vi "CCSaveWorklistResult.vi"(8 "error in (no error)":errorcluster, 9 "patientID":string="C:\\Users\\Simon\\Dropbox\\Medimatic\\ProjectVerLV2011\\tmp.dcm", 10 "index":i32, 11 "Find":refnum<k24>) -> (0 "error out":errorcluster)   [LabVIEW 2013, in "main.lvlib" / "ClearCanvasLibrary.lvlib"]
uses:
  ClearCanvasLibrary.lvlib
  C:/Users/Simon/SkyDrive/LabView/2013/DM2020/DICOM/ClearCanvasNewBuild/ClearCanvas.Dicom.dll
  ClearCanvasNewBuild/ClearCanvas.Dicom.dll
  Globals/DataPathGlobalVariable.vi
  main.lvlib
panel:
  out "Dump":string
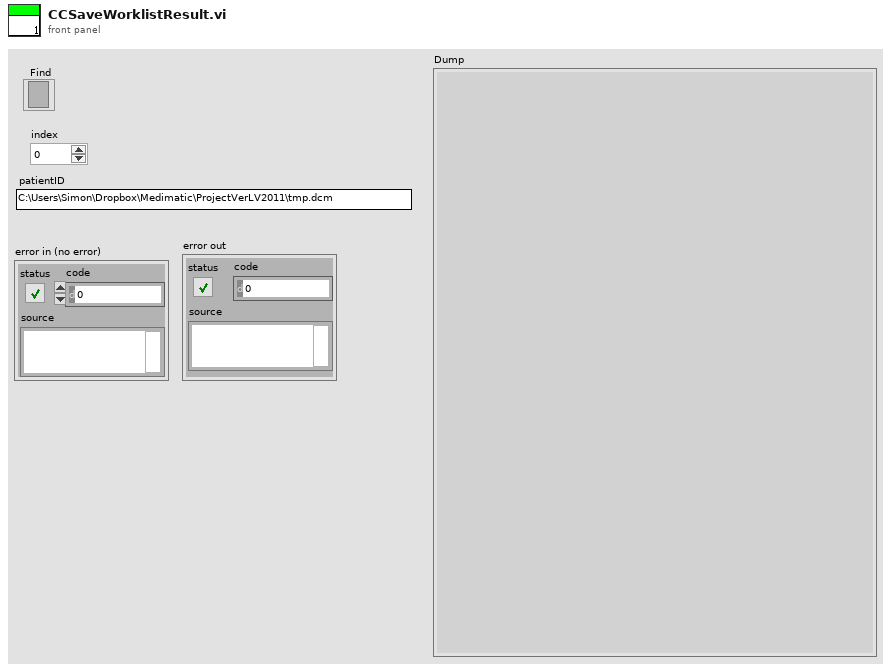
[diagram p1: front panel]
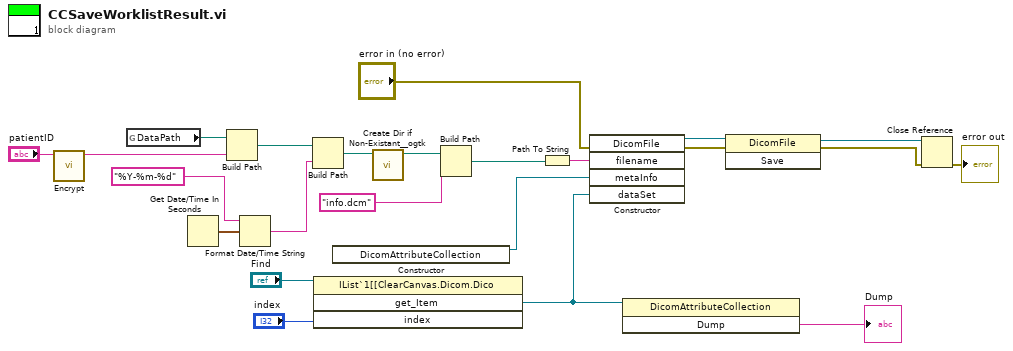
[diagram p0: block diagram]
diagram:
  n1 = call "Encrypt.vi"("Input"="patientID") -> ("Output"=w17:string)  [unwired: 10 in]
  n2 = global read "DataPathGlobalVariable.vi" "DataPath"() -> (w23:path)
  n3 = Get Date/Time In Seconds() -> (seconds since 1Jan1904=w22:timestamp)
  n4 = Build Path(base path=w23, name or relative path=w17) -> (appended path=w20:path)
  n5 = Format Date/Time String(time format string (%c)="%Y-%m-%d", seconds (now)=w22) -> (date/time string=w19:string)  [unwired: 1 in]
  n6 = Build Path(base path=w20, name or relative path=w19) -> (appended path=w6:path)
  n7 = invoke class="IList`1[[ClearCanvas.Dicom.Dico" method="get_Item"(reference="Find", "index"="index") -> ("get_Item"=w4:refnum<k24>)  [unwired: 2 in, 3 out]
  n8 = constructor class="DicomAttributeCollection"() -> (reference out=w3:refnum<k24>)  [unwired: 3 in, 2 out]
  n9 = call <userlib>:"Create Dir if Non-Existant__ogtk.vi"("Directory Path"=w6) -> ("dup Directory Path"=w5:path)  [unwired: 8 in, 2 out]
  n10 = Build Path(base path=w5, name or relative path="info.dcm") -> (appended path=w7:path)
  n11 = Path To String(path=w7) -> (string=w8:string)
  n12 = constructor class="DicomFile"(error in="error in (no error)", "filename"=w8, "metaInfo"=w3, "dataSet"=w4) -> (reference out=w2:refnum<k24>, error out=w1:errorcluster)  [unwired: 2 in, 4 out]
  n13 = invoke class="DicomAttributeCollection" method="Dump"(reference=w4) -> ("Dump"=→"Dump":string)  [unwired: 2 in, 2 out]
  n14 = invoke class="DicomFile" method="Save"(reference=w2, error in=w1) -> (reference out=w10:refnum<k24>, error out=w13:errorcluster)  [unwired: 1 in, 1 out]
  n15 = Close Reference(reference=w10, error in (no error)=w13) -> (error out=→"error out":errorcluster)
